vi "WPI_PotentiometerRefNum Registry Set.vi"(8 "error in (no error)":errorcluster, 9 "Test Mode Only":bool, 10 "refnum name":string="My Pot RefNum", 11 "PotDevRef":T1={"DevStatus"={"status"=FALSE, "code"=0, "source"=""}, "Analog Channel"=enum."Invalid", "Invert Output"=FALSE}) -> (0 "error out":errorcluster, 3 "PotDevRef":T1={"DevStatus"={"status"=FALSE, "code"=0, "source"=""}, "Analog Channel"=enum."Invalid", "Invert Output"=FALSE})   [LabVIEW 2017]
doc: "Sets a reference into a named registry storage. After setting a reference, you can retrieve it by name using the <B>RefNum Registry Get</B>.\nThe <B>Test Mode Only</B> parameter restricts it so Test Mode can use the reference, but other code cannot get the refnum and modify the I/O."
uses:
  <vilib>/Rock Robotics/WPI/Potentiometer/WPI_PotentiometerDevRef.ctl
  <vilib>/Rock Robotics/SystemInterfaces/AI/FPGA_AIChannel.ctl
  <vilib>/Rock Robotics/WPI/Utilities/Refnum Registry Operation.ctl
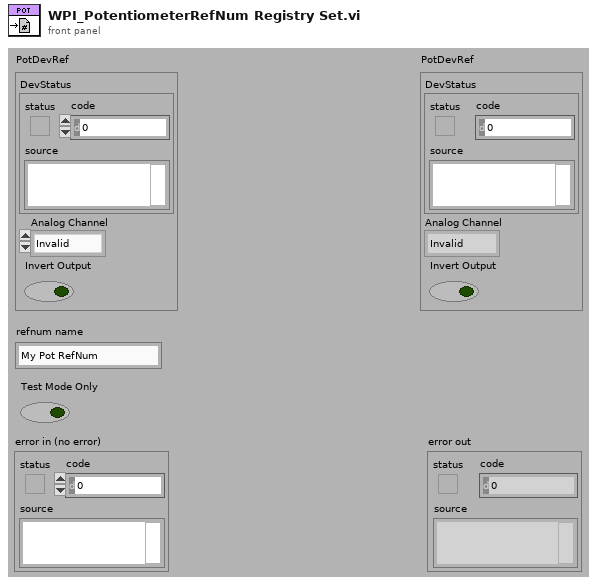
[diagram p1: front panel]
types:
  T1 = typedef "WPI_PotentiometerDevRef.ctl" = cluster{"DevStatus":errorcluster, "Analog Channel":T2, "Invert Output":bool}
  T2 = typedef "FPGA_AIChannel.ctl" = enum8{"AI 0", "AI 1", "AI 2", "AI 3", "AI MXP 0", "AI MXP 1", "AI MXP 2", "AI MXP 3", "Invalid"}
  T3 = typedef "Refnum Registry Operation.ctl" = enum16{"set", "get", "delete", "get all names", "read name"}
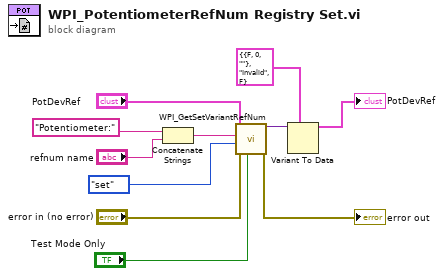
[diagram p0: block diagram]
diagram:
  n1 = Concatenate Strings("Potentiometer:", "refnum name") -> (w11:string)
  n2 = call <vilib>:"WPI_GetSetVariantRefNum.vi"("Test Mode Only"="Test Mode Only", "error in (no error)"="error in (no error)", "Operation"=Refnum_Registry_Operation."set" ("menu"), "refnum name"=w11, "DevRef"="PotDevRef") -> ("error out"=→"error out":errorcluster, "DevRef"=w9:variant)  [unwired: 4 in, 1 out]
  n3 = Variant To Data(type=T1 {"DevStatus"={"status"=FALSE, "code"=0, "source"=""}, "Analog Channel"=enum."Invalid", "Invert Output"=FALSE} ("PotDevRef"), Variant=w9) -> (data=→"PotDevRef":T1)  [unwired: 1 in, 1 out]
